vi "Analog_Output_2.vi"() -> ()   [LabVIEW 2019]
uses:
  <vilib>/DAQmx/write.llb/DAQmx Write (Analog Wfm 1Chan NSamp).vi
  <vilib>/DAQmx/create/channels.llb/DAQmx Create Channel (AO-Voltage-Basic).vi
  <vilib>/DAQmx/configure/timing.llb/DAQmx Timing (Use Waveform).vi
  <vilib>/DAQmx/miscellaneous.llb/DAQmx Fill In Error Info.vi
  <vilib>/measure/NI_MABase.lvlib
panel:
  in  "physical channels":tag caption="물리적 채널"
  out "웨이브폼 그래프":waveform(dbl)(graph)
  in  "amplitude":dbl=1.0 caption="진폭" format="%0.2p"
  in  "frequency":dbl=10.0 caption="주파수" format="%0.2p"
  in  "sampling info":cluster{"Fs":dbl, "#s":dbl}={"Fs"=1000.0, "#s"=1000.0} caption="샘플링 정보" {"Fs" format="%.2p"}
  in  "정지버튼":bool
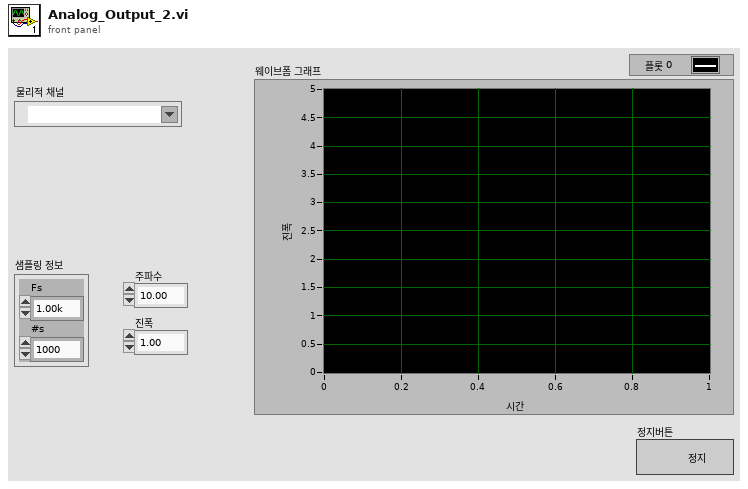
[diagram p1: front panel]
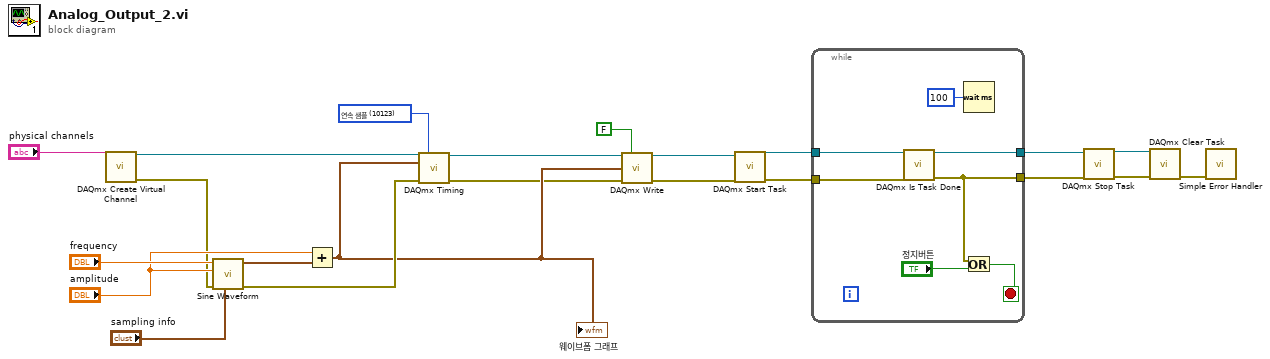
[diagram p0: block diagram]
diagram:
  w15 = 10123 items=["유한 샘플"=10178, "연속 샘플"=10123, "하드웨어 타이밍에 의한 단일 포인트"=12522] ("sample mode")
  n1 = call-poly <vilib>:"DAQmx Create Virtual Channel.vi"("physical channels"="physical channels") -> ("task out"=w9:refnum<k21>, "error out"=w10:errorcluster)  [unwired: 13 in]
  n2 = call <vilib>:"Sine Waveform.vi"("sampling info"="sampling info", "error in (no error)"=w10, "amplitude"="amplitude", "frequency"="frequency") -> ("error out"=w8:errorcluster, "signal out"=w12:waveform(dbl))  [unwired: 6 in]
  n3 = Add(x="amplitude", y=w12) -> (x+y=w7:waveform(dbl))
  "웨이브폼 그래프" <- w7
  n4 = call-poly <vilib>:"DAQmx Timing.vi"("task/channels in"=w9, "sample mode"=w15, "waveform"=w7, "error in"=w8) -> ("task out"=w2:refnum<k21>, "error out"=w1:errorcluster)  [unwired: 10 in]
  n5 = call-poly <vilib>:"DAQmx Write.vi"("task/channels in"=w2, "auto start"=FALSE, "data"=w7, "error in"=w1) -> ("task out"=w5:refnum<k21>, "error out"=w6:errorcluster)  [unwired: 9 in, 1 out]
  n6 = call <vilib>:"DAQmx Start Task.vi"("task/channels in"=w5, "error in"=w6) -> ("task out"=w22:refnum<k21>, "error out"=w21:errorcluster)  [unwired: 12 in]
  n7 = while {
    tunnel: w22 -> [w29]
    tunnel: w21 -> [w28]
    tunnel: [w24] -> w20
    tunnel: [w25] -> w19
    stop <- w27 stop-if-true
    n8 = call <vilib>:"DAQmx Is Task Done.vi"("task/channels in"=w29, "error in"=w28) -> ("task out"=w24:refnum<k21>, "error out"=w25:errorcluster)  [unwired: 11 in, 1 out]
    n9 = Wait (ms)(milliseconds to wait=u32 100 ("대기 시간 (ms)")) -> ()  [unwired: 1 out]
    n10 = Or(x=w25, y="정지버튼") -> (x .or. y?=w27:bool)
  }
  n11 = call <vilib>:"DAQmx Stop Task.vi"("task/channels in"=w20, "error in"=w19) -> ("task out"=w18:refnum<k21>, "error out"=w17:errorcluster)  [unwired: 12 in]
  n12 = call <vilib>:"DAQmx Clear Task.vi"("task in"=w18, "error in"=w17) -> ("error out"=w16:errorcluster)  [unwired: 13 in]
  n13 = call <vilib>:"Simple Error Handler.vi"("error in (no error)"=w16) -> ()  [unwired: 4 in, 5 out]
